vi "Query Capabilities (Sample).vi"(0 "VISA resource name":refnum<visa-resource-name>, 5 "Absolute Maximums (T)":bool=TRUE, 11 "error in (no error)":errorcluster) -> (4 "VISA resource name out":refnum<visa-resource-name>, 6 "Minimum (Hz)":dbl, 8 "Maximum (Hz)":dbl, 10 "Points":u32 max=12 step=1, 15 "error out":errorcluster)   [LabVIEW 2020, in "NH Research Regenerative Test Series.lvlib"]
doc: "This will query the absolute minimum and maximum frequency for measuring samples and the absolute maximum legal values for the number of samples."
uses:
  NH Research Regenerative Test Series.lvlib
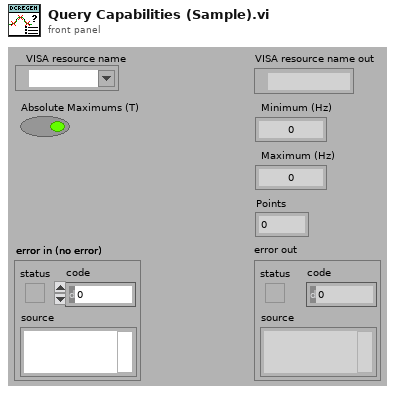
[diagram p1: front panel]
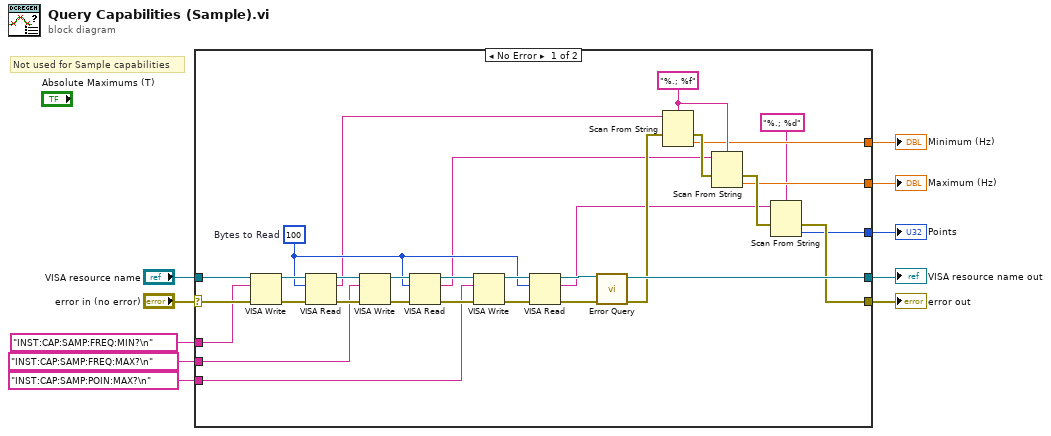
[diagram p0: block diagram]
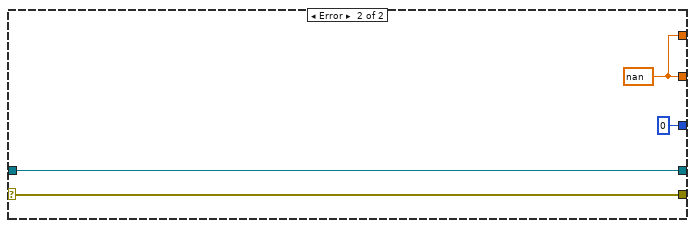
[diagram p2: hidden frame]
diagram:
  # "Not used for Sample capabilities"
  n1 = case shown="No Error" "error in (no error)" {
    selector: "error in (no error)" -> [w39 w45]
    tunnel: [w19 w45] -> w9
    tunnel: [w37 w44] -> w7
    tunnel: "VISA resource name" -> [w38 w44]
    tunnel: "INST:CAP:SAMP:FREQ:MIN?\n" ("write buffer") -> [w29 _]
    tunnel: "INST:CAP:SAMP:FREQ:MAX?\n" ("write buffer") -> [w28 _]
    tunnel: "INST:CAP:SAMP:POIN:MAX?\n" ("write buffer") -> [w27 _]
    tunnel: [w18 w43] -> w2
    tunnel: [w17 u32 0] -> w1
    tunnel: [w12 w43] -> w3
    frame No Error {
      w13 = "%.; %f" ("format string")
      w24 = u32 100  # Bytes to Read
      n2 = VISA Write(VISA resource name=w38, write buffer=w29, error in (no error)=w39) -> (VISA resource name out=w40:refnum<visa-resource-name>, error out=w41:errorcluster)  [unwired: 1 out]
      n3 = VISA Read(VISA resource name=w40, byte count=w24, error in (no error)=w41) -> (VISA resource name out=w26:refnum<visa-resource-name>, read buffer=w16:string, error out=w31:errorcluster)  [unwired: 1 out]
      n4 = VISA Write(VISA resource name=w26, write buffer=w28, error in (no error)=w31) -> (VISA resource name out=w34:refnum<visa-resource-name>, error out=w35:errorcluster)  [unwired: 1 out]
      n5 = VISA Read(VISA resource name=w34, byte count=w24, error in (no error)=w35) -> (VISA resource name out=w25:refnum<visa-resource-name>, read buffer=w15:string, error out=w30:errorcluster)  [unwired: 1 out]
      n6 = VISA Write(VISA resource name=w25, write buffer=w27, error in (no error)=w30) -> (VISA resource name out=w32:refnum<visa-resource-name>, error out=w33:errorcluster)  [unwired: 1 out]
      n7 = VISA Read(VISA resource name=w32, byte count=w24, error in (no error)=w33) -> (VISA resource name out=w22:refnum<visa-resource-name>, read buffer=w14:string, error out=w23:errorcluster)  [unwired: 1 out]
      n8 = call "Error Query.vi"("VISA resource name"=w22, "error in (no error)"=w23) -> ("VISA resource name out"=w37:refnum<visa-resource-name>, "error out"=w36:errorcluster)  [unwired: 10 in, 2 out]
      n9 = Scan From String(format string=w13, input string=w16, error in=w36) -> (error out=w21:errorcluster, output 1=w12:dbl)  [unwired: 2 in, 2 out]
      n10 = Scan From String(format string=w13, input string=w15, error in=w21) -> (error out=w20:errorcluster, output 1=w18:dbl)  [unwired: 2 in, 2 out]
      n11 = Scan From String(format string="%.; %d", input string=w14, error in=w20) -> (error out=w19:errorcluster, output 1=w17:i32)  [unwired: 2 in, 2 out]
    }
    frame Error {
      w43 = nan
    }
  }
  "error out" <- w9
  "VISA resource name out" <- w7
  "Minimum (Hz)" <- w3
  "Maximum (Hz)" <- w2
  "Points" <- w1
